vi "ep_Replace Ranges Core.vi"(5 "waveform":waveform(dbl), 7 "full-range RMS values":dbl, 8 "error in":errorcluster, 10 "current ranges (multiline) in":T1[](array[typedef]), 11 "voltage ranges (multiline) in":T1[](array[typedef])) -> (0 "error out":errorcluster, 2 "current ranges (multiline) out":T1[](array[typedef]), 3 "voltage ranges (multiline) out":T1[](array[typedef]))   [LabVIEW 2014, in "NI_EP_Power Quality.lvlib"]
uses:
  <vilib>/addons/Electrical Power/PQ/NI_EP_Power Quality.lvlib
  <vilib>/addons/Electrical Power/PQ/Common/Controls/ep_Channel Ranges.ctl
  <vilib>/addons/Electrical Power/PQ/Common/Controls/ep_AI Data Channel.ctl
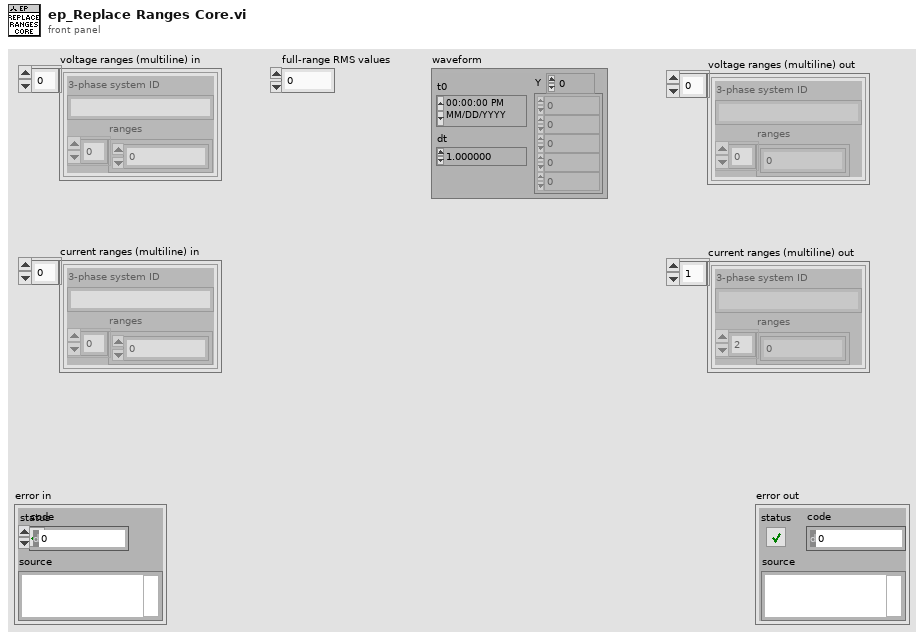
[diagram p1: front panel]
types:
  T1 = typedef "NI_EP_Power Quality.lvlib/ep_Channel Ranges.ctl" = cluster{"3-phase system ID":string, "ranges":dbl[]}
  T2 = typedef "NI_EP_Power Quality.lvlib/ep_AI Data Channel.ctl" = enum16{"Voltage Phase A (L1)", "Voltage Phase B (L2)", "Voltage Phase C (L3)", "Voltage Phase N (Neutral)", "Current Phase A (L1)", "Current Phase B (L2)", "Current Phase C (L3)", "Current Phase N (Neutral)"}
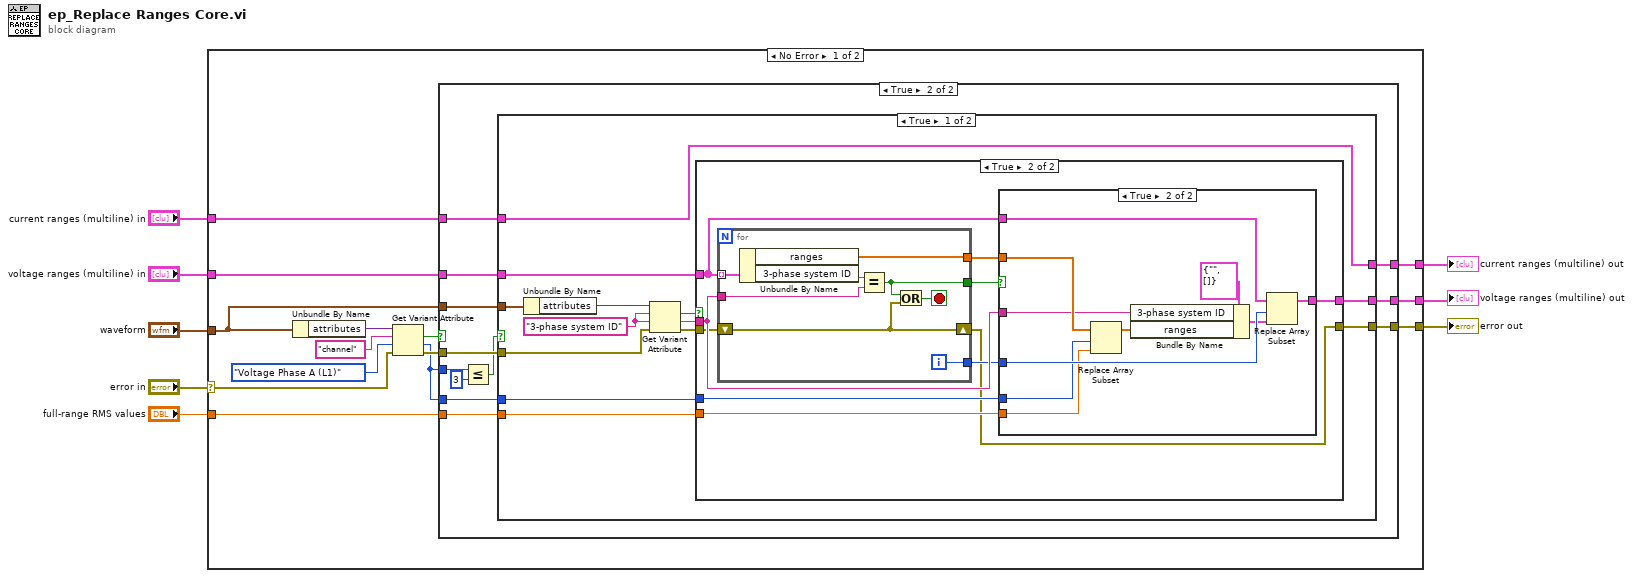
[diagram p0: block diagram]
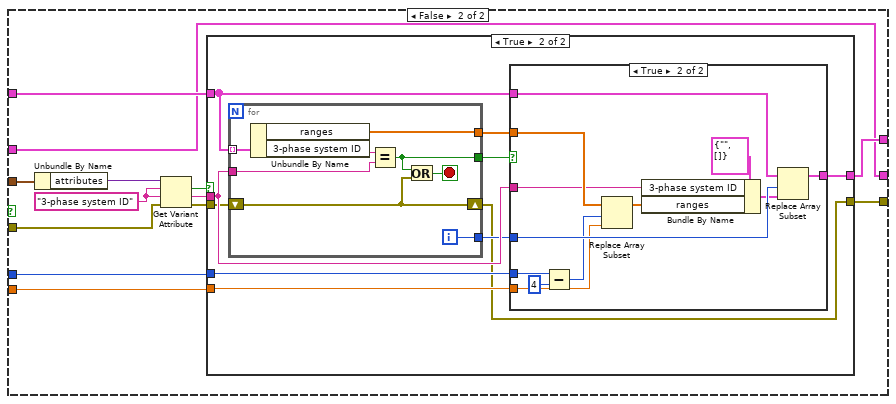
[diagram p5: hidden frame]
diagram:
  n1 = case shown="No Error" "error in" {
    selector: "error in" -> [w12 w128]
    tunnel: "voltage ranges (multiline) in" -> [w22 _]
    tunnel: "current ranges (multiline) in" -> [w21 _]
    tunnel: "waveform" -> [w14 _]
    tunnel: "full-range RMS values" -> [w19 _]
    tunnel: [w20 w128] -> w3
    tunnel: [w18 _] -> w2
    tunnel: [w17 _] -> w1
    frame No Error {
      n2 = Unbundle By Name(w14) -> ("attributes"=w16:variant)
      n3 = Get Variant Attribute(Variant=w16, name="channel", default value (empty Variant)=ep_AI_Data_Channel."Voltage Phase A (L1)" ("channel"), error in=w12) -> (found=w10:bool, value=w9:T2, error out=w11:errorcluster)  [unwired: 1 out]
      n4 = case shown="True" w10 {
        tunnel: w11 -> [w25 w37]
        tunnel: w22 -> [w23 w36]
        tunnel: w21 -> [w24 w35]
        tunnel: w14 -> [_ w34]
        tunnel: w19 -> [_ w33]
        tunnel: [w25 w32] -> w20
        tunnel: [w23 w31] -> w18
        tunnel: [w24 w30] -> w17
        tunnel: w9 -> [_ w28]
        tunnel: w9 -> [_ w26]
        frame False {
        }
        frame True {
          n5 = Less Or Equal?(x=w28, y=3) -> (x <= y?=w29:bool)
          n6 = case shown="True" w29 {
            tunnel: w34 -> [w44 w89]
            tunnel: w36 -> [w45 w82]
            tunnel: w37 -> [w48 w92]
            tunnel: [w43 w88] -> w32
            tunnel: w35 -> [w39 w84]
            tunnel: w33 -> [w42 w87]
            tunnel: [w40 w82] -> w31
            tunnel: [w39 w83] -> w30
            tunnel: w26 -> [w38 w85]
            frame True {
              w49 = "3-phase system ID" ("name")
              n7 = Unbundle By Name(w44) -> ("attributes"=w50:variant)
              n8 = Get Variant Attribute(Variant=w50, name=w49, default value (empty Variant)=w49, error in=w48) -> (found=w41:bool, value=w47:string, error out=w46:errorcluster)  [unwired: 1 out]
              n9 = case shown="True" w41 {
                tunnel: w47 -> [_ w60]
                tunnel: w46 -> [w52 w59]
                tunnel: w45 -> [w51 w58]
                tunnel: [w52 w53] -> w43
                tunnel: w42 -> [_ w56]
                tunnel: [w51 w55] -> w40
                tunnel: w38 -> [_ w54]
                frame False {
                }
                frame True {
                  n10 = for {
                    tunnel: w58 -> [w81] mode=indexing
                    tunnel: w60 -> [w79]
                    shift-right: [w78] -> w53
                    shift-left: w59 -> [w78]
                    tunnel: [w74] -> w62
                    tunnel: [w76] -> w61
                    tunnel: [w75] -> w57
                    i -> [w75]
                    stop <- w77 stop-if-true
                    n11 = Unbundle By Name(w81) -> ("ranges"=w76:dbl[], "3-phase system ID"=w80:string)
                    n12 = Equal?(x=w80, y=w79) -> (x = y?=w74:bool)
                    n13 = Or(x=w74, y=w78) -> (x .or. y?=w77:bool)
                  }
                  n14 = case shown="True" w62 {
                    tunnel: w61 -> [_ w73]
                    tunnel: w60 -> [_ w72]
                    tunnel: w58 -> [w63 w71]
                    tunnel: w57 -> [_ w70]
                    tunnel: w56 -> [_ w69]
                    tunnel: [w63 w68] -> w55
                    tunnel: w54 -> [_ w64]
                    frame False {
                    }
                    frame True {
                      n15 = Replace Array Subset(array=w73, new element=w69, index=w64) -> (w67:dbl[])
                      n16 = Bundle By Name(cluster=T1 {"3-phase system ID"="", "ranges"=[]} ("voltage ranges (multiline)"), "3-phase system ID"=w72, "ranges"=w67) -> (w65:T1)
                      n17 = Replace Array Subset(array=w71, new element=w65, index=w70) -> (w68:T1[])
                    }
                  }
                }
              }
            }
            frame False {
              w93 = "3-phase system ID" ("name")
              n18 = Unbundle By Name(w89) -> ("attributes"=w94:variant)
              n19 = Get Variant Attribute(Variant=w94, name=w93, default value (empty Variant)=w93, error in=w92) -> (found=w86:bool, value=w91:string, error out=w90:errorcluster)  [unwired: 1 out]
              n20 = case shown="True" w86 {
                tunnel: w91 -> [_ w104]
                tunnel: w90 -> [w96 w103]
                tunnel: [w96 w98] -> w88
                tunnel: w87 -> [_ w101]
                tunnel: [w95 w100] -> w83
                tunnel: w85 -> [_ w99]
                tunnel: w84 -> [w95 w97]
                frame False {
                }
                frame True {
                  n21 = for {
                    tunnel: w97 -> [w127] mode=indexing
                    tunnel: w104 -> [w125]
                    shift-right: [w124] -> w98
                    shift-left: w103 -> [w124]
                    tunnel: [w120] -> w106
                    tunnel: [w122] -> w105
                    tunnel: [w121] -> w102
                    i -> [w121]
                    stop <- w123 stop-if-true
                    n22 = Unbundle By Name(w127) -> ("ranges"=w122:dbl[], "3-phase system ID"=w126:string)
                    n23 = Equal?(x=w126, y=w125) -> (x = y?=w120:bool)
                    n24 = Or(x=w120, y=w124) -> (x .or. y?=w123:bool)
                  }
                  n25 = case shown="True" w106 {
                    tunnel: w105 -> [_ w119]
                    tunnel: w104 -> [_ w118]
                    tunnel: w97 -> [w107 w117]
                    tunnel: w102 -> [_ w116]
                    tunnel: w101 -> [_ w115]
                    tunnel: [w107 w114] -> w100
                    tunnel: w99 -> [_ w110]
                    frame False {
                    }
                    frame True {
                      n26 = Subtract(x=w110, y=4) -> (x-y=w109:i32)
                      n27 = Replace Array Subset(array=w119, new element=w115, index=w109) -> (w113:dbl[])
                      n28 = Bundle By Name(cluster=T1 {"3-phase system ID"="", "ranges"=[]} ("voltage ranges (multiline)"), "3-phase system ID"=w118, "ranges"=w113) -> (w111:T1)
                      n29 = Replace Array Subset(array=w117, new element=w111, index=w116) -> (w114:T1[])
                    }
                  }
                }
              }
            }
          }
        }
      }
    }
    frame Error {
    }
  }
  "error out" <- w3
  "current ranges (multiline) out" <- w1
  "voltage ranges (multiline) out" <- w2
